vi "TL_read_next_task_TDMS.vi"(3 "error in":errorcluster, 5 "Reset":bool) -> (0 "error out":errorcluster, 2 "task":T1)   [LabVIEW 2015]
uses:
  CONTROLS/Q_main_element.ctl
  GLOBAL/Global_ABORT.vi
  GLOBAL/Global_MAIN.vi
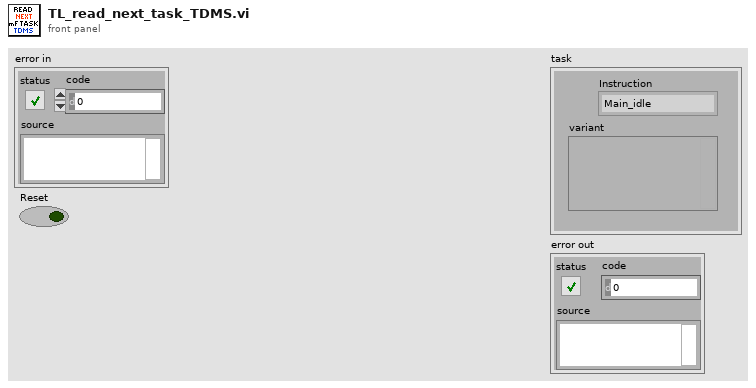
[diagram p1: front panel]
types:
  T1 = typedef "Q_main_element.ctl" = cluster{"variant":variant, "Instruction":enum16{"Main_idle", "Main_initialize", "Main_initialize_TDMS", "Main_initialize_Queue", "Main_error", "Main_DAQ_initialization_results", "Main_ASI_initialization_results", "Main_Piezo_initialization_results", "Main_Valve_initialization_results", "Main_Pump_initialization_results", "Main_CAMERA_initialization_results", "Main_DAQ_error", "Main_ASI_error", "Main_Piezo_error", "Main_CAMERA_error", "Main_Valve_error", "Main_Pump_error", "Main_start_acquiring", "Main_not_acquiring", "Main_acquiring", "Main_stop_acquiring", "Main_change_exposure", "Main_change_z_scan_parameters", "Main_define_ROI", "Main_define_mosaic", "Main_read_kinetic_time", "Main_cooler", "Main_read_temperature", "Main_save_XY", "Main_load_XY", "Main_discard_XY", "Main_move_to_XY", "Main_measure_QPD", "Main_autofocus_calibration", "Main_save_PID", "Main_change_H_valve_position", "Main_two_way_valve", "Main_save_movie", "Main_init_single_scan", "Main_single_scan", "Main_stop_single_scan", "Main_merFISH_illumination_parameters", "Main_merFISH_buffer_probe_list", "Main_merFISH_injections_procedure", "Main_merFISH_save_setpoint", "Main_merFISH_DAPI_parameters", "Main_merFISH_Brightfield_parameters", "Main_merFISH_save_embryo_ROI", "Main_merFISH_init", "Main_merFISH_resume", "Main_merFISH_start_autofocus", "Main_merFISH_open_close_valve_merFISH", "Main_merFISH_open_close_valve_photobleaching", "Main_merFISH_hybridization", "Main_merFISH_move_to_ROI", "Main_merFISH_wait_stabilization", "Main_merFISH_scan_laser", "Main_merFISH_scan_brightfield", "Main_merFISH_photobleaching_injection", "Main_merFISH_photobleaching", "Main_merFISH_save", "Main_merFISH_send_email", "Main_merFISH_close", "Main_TL_define_parameters", "Main_TL_reset_parameters", "Main_TL_init", "Main_TL_start_autofocus", "Main_TL_move_to_ROI", "Main_TL_wait_for_stabilization", "Main_TL_scan", "Main_TL_wait_cycle_end", "Main_TL_close", "Main_STOP"}}
  T2 = enum16{"open", "open or create", "create or replace", "create", "open (read-only)"}
  T3 = enum16{"Main_idle", "Main_initialize", "Main_initialize_TDMS", "Main_initialize_Queue", "Main_error", "Main_DAQ_initialization_results", "Main_ASI_initialization_results", "Main_Piezo_initialization_results", "Main_Valve_initialization_results", "Main_Pump_initialization_results", "Main_CAMERA_initialization_results", "Main_DAQ_error", "Main_ASI_error", "Main_Piezo_error", "Main_CAMERA_error", "Main_Valve_error", "Main_Pump_error", "Main_start_acquiring", "Main_not_acquiring", "Main_acquiring", "Main_stop_acquiring", "Main_change_exposure", "Main_change_z_scan_parameters", "Main_define_ROI", "Main_define_mosaic", "Main_read_kinetic_time", "Main_cooler", "Main_read_temperature", "Main_save_XY", "Main_load_XY", "Main_discard_XY", "Main_move_to_XY", "Main_measure_QPD", "Main_autofocus_calibration", "Main_save_PID", "Main_change_H_valve_position", "Main_two_way_valve", "Main_save_movie", "Main_init_single_scan", "Main_single_scan", "Main_stop_single_scan", "Main_merFISH_illumination_parameters", "Main_merFISH_buffer_probe_list", "Main_merFISH_injections_procedure", "Main_merFISH_save_setpoint", "Main_merFISH_DAPI_parameters", "Main_merFISH_Brightfield_parameters", "Main_merFISH_save_embryo_ROI", "Main_merFISH_init", "Main_merFISH_resume", "Main_merFISH_start_autofocus", "Main_merFISH_open_close_valve_merFISH", "Main_merFISH_open_close_valve_photobleaching", "Main_merFISH_hybridization", "Main_merFISH_move_to_ROI", "Main_merFISH_wait_stabilization", "Main_merFISH_scan_laser", "Main_merFISH_scan_brightfield", "Main_merFISH_photobleaching_injection", "Main_merFISH_photobleaching", "Main_merFISH_save", "Main_merFISH_send_email", "Main_merFISH_close", "Main_TL_define_parameters", "Main_TL_reset_parameters", "Main_TL_init", "Main_TL_start_autofocus", "Main_TL_move_to_ROI", "Main_TL_wait_for_stabilization", "Main_TL_scan", "Main_TL_wait_cycle_end", "Main_TL_close", "Main_STOP"}
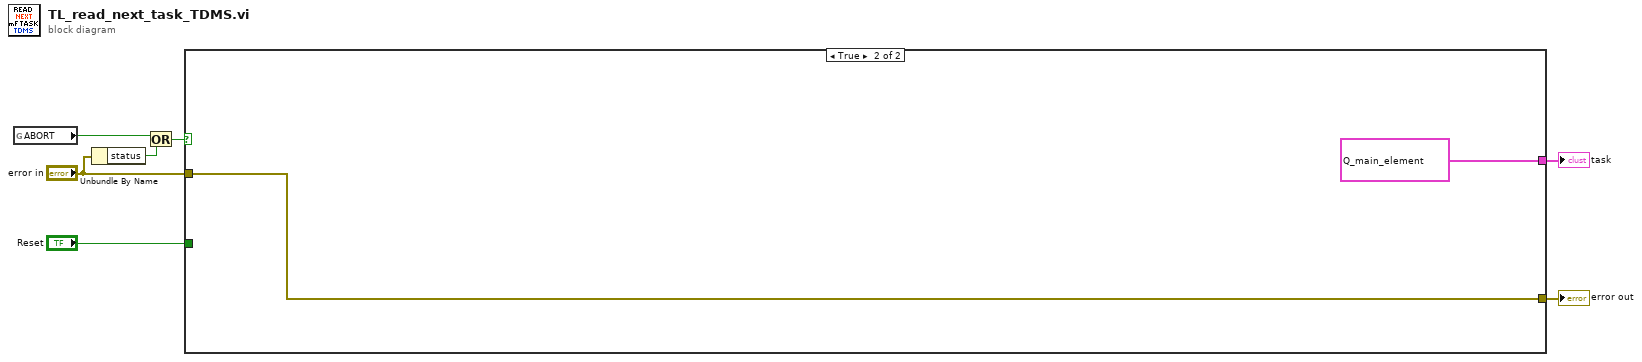
[diagram p0: block diagram]
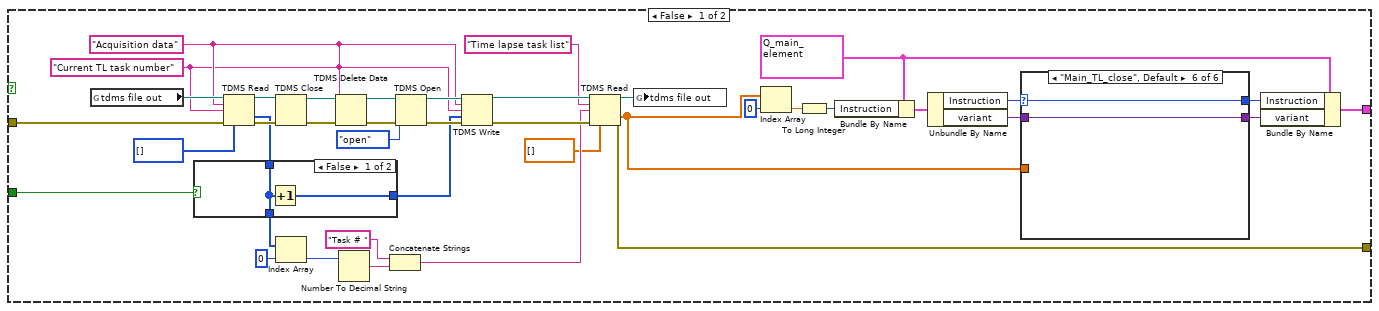
[diagram p2: hidden frame]
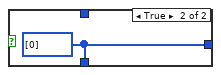
[diagram p3: hidden frame]
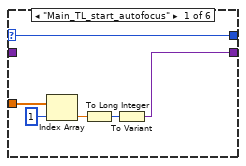
[diagram p4: hidden frame]
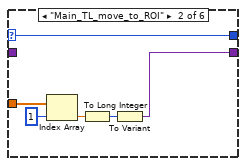
[diagram p5: hidden frame]
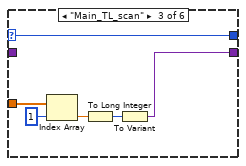
[diagram p6: hidden frame]
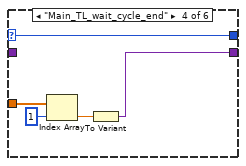
[diagram p7: hidden frame]
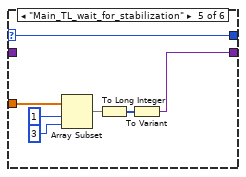
[diagram p8: hidden frame]
diagram:
  n1 = global read "Global_ABORT.vi" "ABORT"() -> (w7:bool)
  n2 = Unbundle By Name("error in") -> ("status"=w6:bool)
  n3 = Or(x=w7, y=w6) -> (x .or. y?=w4:bool)
  n4 = case shown="True" w4 {
    tunnel: "error in" -> [w15 w83]
    tunnel: [w14 T1 {"variant"=variant, "Instruction"=enum."Main_TL_close"} ("element")] -> w3
    tunnel: [w13 w83] -> w2
    tunnel: "Reset" -> [w11 _]
    frame False {
      w18 = T1 {"variant"=variant, "Instruction"=enum."Main_idle"} ("element")
      w36 = "Current TL task number" ("group name in")
      w37 = "Acquisition data" ("group name in")
      n5 = global read "Global_MAIN.vi" "tdms file out"() -> (w47:refnum<k34>)
      n6 = TDMS Read(0:w47, 5:w37, 7:w36, 11:w15, 12:u32[] [] ("appended array")) -> (4:w27:refnum<k34>, 10:w34:u32[], 15:w40:errorcluster)  [unwired: 3 in, 3 out]
      n7 = case shown="False" w11 {
        tunnel: w34 -> [w48 _]
        tunnel: [w49 w50] -> w33
        tunnel: [w48 w50] -> w10
        frame False {
          n8 = Increment(x=w48) -> (x+1=w49:u32[])
        }
        frame True {
          w50 = u32[] [0]
        }
      }
      n9 = TDMS Close(8:w40, 11:w27) -> (0:w41:errorcluster, 3:w42:path)
      n10 = Index Array(array=w10, index=0) -> (element=w30:u32)
      n11 = TDMS Delete Data(8:w41, 9:w36, 10:w37, 11:w42) -> (0:w44:errorcluster, 3:w45:path)  [unwired: 3 in]
      n12 = Number To Decimal String(number=w30) -> (decimal integer string=w31:string)  [unwired: 1 in]
      n13 = Concatenate Strings("Task # " ("string"), w31) -> (w25:string)
      n14 = TDMS Open(8:w44, 10:T2."open" ("operation (0:open)"), 11:w45) -> (0:w39:errorcluster, 3:w38:refnum<k34>)  [unwired: 4 in]
      n15 = TDMS Write(0:w38, 5:w37, 7:w36, 9:w33, 11:w39) -> (4:w29:refnum<k34>, 15:w28:errorcluster)  [unwired: 1 in, 2 out]
      n16 = TDMS Read(0:w29, 5:"Time lapse task list" ("group name in (Untitled)"), 7:w25, 11:w28, 12:dbl[] []) -> (4:w12:refnum<k34>, 10:w19:dbl[], 15:w13:errorcluster)  [unwired: 3 in, 3 out]
      n17 = global write "Global_MAIN.vi" "tdms file out"(w12) -> ()
      n18 = Index Array(array=w19, index=0) -> (element=w23:dbl)
      n19 = To Long Integer(number=w23) -> (32bit integer=w8:i32)
      n20 = Bundle By Name(cluster=w18, "Instruction"=w8) -> (w22:T1)
      n21 = Unbundle By Name(w22) -> ("Instruction"=w21:T3, "variant"=w20:variant)
      n22 = case shown="\"Main_TL_close\", Default" w21 {
        selector: w21 -> [w56 w62 w68 w73 w80 w82]
        tunnel: w20 -> [_ _ _ _ _ w81]
        tunnel: [w56 w62 w68 w73 w80 w82] -> w17
        tunnel: [w52 w58 w64 w69 w79 w81] -> w16
        tunnel: w19 -> [w55 w61 w67 w72 w78 _]
        frame "Main_TL_start_autofocus" {
          n23 = Index Array(array=w55, index=1) -> (element=w53:dbl)
          n24 = To Long Integer(number=w53) -> (32bit integer=w51:i32)
          n25 = To Variant(anything=w51) -> (Variant=w52:variant)
        }
        frame "Main_TL_move_to_ROI" {
          n26 = Index Array(array=w61, index=1) -> (element=w59:dbl)
          n27 = To Long Integer(number=w59) -> (32bit integer=w57:i32)
          n28 = To Variant(anything=w57) -> (Variant=w58:variant)
        }
        frame "Main_TL_scan" {
          n29 = Index Array(array=w67, index=1) -> (element=w65:dbl)
          n30 = To Long Integer(number=w65) -> (32bit integer=w63:i32)
          n31 = To Variant(anything=w63) -> (Variant=w64:variant)
        }
        frame "Main_TL_wait_cycle_end" {
          n32 = Index Array(array=w72, index=1) -> (element=w70:dbl)
          n33 = To Variant(anything=w70) -> (Variant=w69:variant)
        }
        frame "Main_TL_wait_for_stabilization" {
          n34 = Array Subset(array=w78, index=1, length=3) -> (w75:dbl[])
          n35 = To Long Integer(number=w75) -> (32bit integer=w74:i32[])
          n36 = To Variant(anything=w74) -> (Variant=w79:variant)
        }
        frame "Main_TL_close", Default {
        }
      }
      n37 = Bundle By Name(cluster=w18, "Instruction"=w17, "variant"=w16) -> (w14:T1)
    }
    frame True {
    }
  }
  "task" <- w3
  "error out" <- w2
